vi "BRig_dataLC_ENL2_First_Count_l1.vi"() -> (2 "output_ENL2_First_Count":i32)   [LabVIEW 2014]
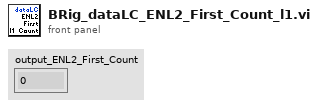
[diagram p1: front panel]
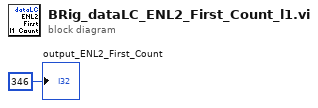
[diagram p0: block diagram]
diagram:
  "output_ENL2_First_Count" <- 346 ("output_iBlock")
